vi "RT-FPGA引用全局.vi"() -> ()   [LabVIEW 2013]
panel:
  out "FPGA VI引用输出":refnum<k20> caption="RT-FPGA引用"
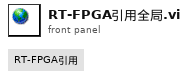
[diagram p1: front panel]
diagram:
